vi "o3 49i Serial Data Recording & DECADEv3.1.vi"() -> ()   [LabVIEW 2014]
uses:
  <vilib>/Platform/TimedLoop/XDataNode/timing_clust.ctl
  <vilib>/Platform/TimedLoop/XDataNode/nitl_modes.ctl
  <vilib>/Platform/TimedLoop/XDataNode/wakeup.ctl
  C:/Program Files (x86)/National Instruments/LabVIEW 2014/examples/Data Communication/Network Streams/Simple Network Streams/support/Network Stream Command.ctl
  <vilib>/Utility/error.llb/whitespace.ctl
  <vilib>/Instr/_visa.llb/VISA Configure Serial Port (Instr).vi
  <vilib>/Utility/tcp.llb/UDP Multicast Write-Only Open.vi
  <vilib>/platform/TimedLoop/XDataNode/XDataNode.xnode
  <vilib>/Platform/TimedLoop/XDataNode/XDNodeRunTimeDep.lvlib
panel:
  out "Stop File Write":bool
  out "Default file name":string
  out "error out":errorcluster
  out "V6":bool
  in  "Clear Display\nErrors":bool
  out "Data Processing":bool
  out "Serial Visa Error":errorcluster
  out "SEPTIC TCP Error Out":errorcluster
  out "TCP packet\nSend to SEPTIC":bool
  out "UDP Time Stamp Offset":i32=1
  out "Data Array":string[](array[string])
  out "UDP packet \nstatus":bool
  out "UDP_Out_Error":errorcluster
  out "FISH TCP Error Out":errorcluster
  out "TCP packet\nSend to FISH":bool
  out "TCP Binary Packet":string
  out "Scan from String Error Counter\nfrom process loop":i32
  out "Read Error Counter\nfrom process loop":i32
  in  "milliseconds to wait":u32=330
  in  "ID":string="»"
  in  "VISA resource name":refnum<visa-resource-name>="ASRL6::INSTR"
  out "Data In Array":string[](array[string])
  out "UDP_ASCII_Out":string
  out "UDP_Pack_num":u32
  out "Flight Number":string
  in  "ue9LJ temp":u16
  out "Data String":string
  out "Internal packet":string[](array[string])
  out "RAW DATA":string
  in  "stop":bool
  out "Number of Send & Read Error\nfrom Acquire Loop":i32
  out "Command In":string
  # "o3_conc"
  # "Bench_temp"
  # "pressure"
  # "cell_a_nt"
  # "cell_b_int"
  # "flow_a"
  # "flow_b"
  # "lamp_temp"
  # "flags"
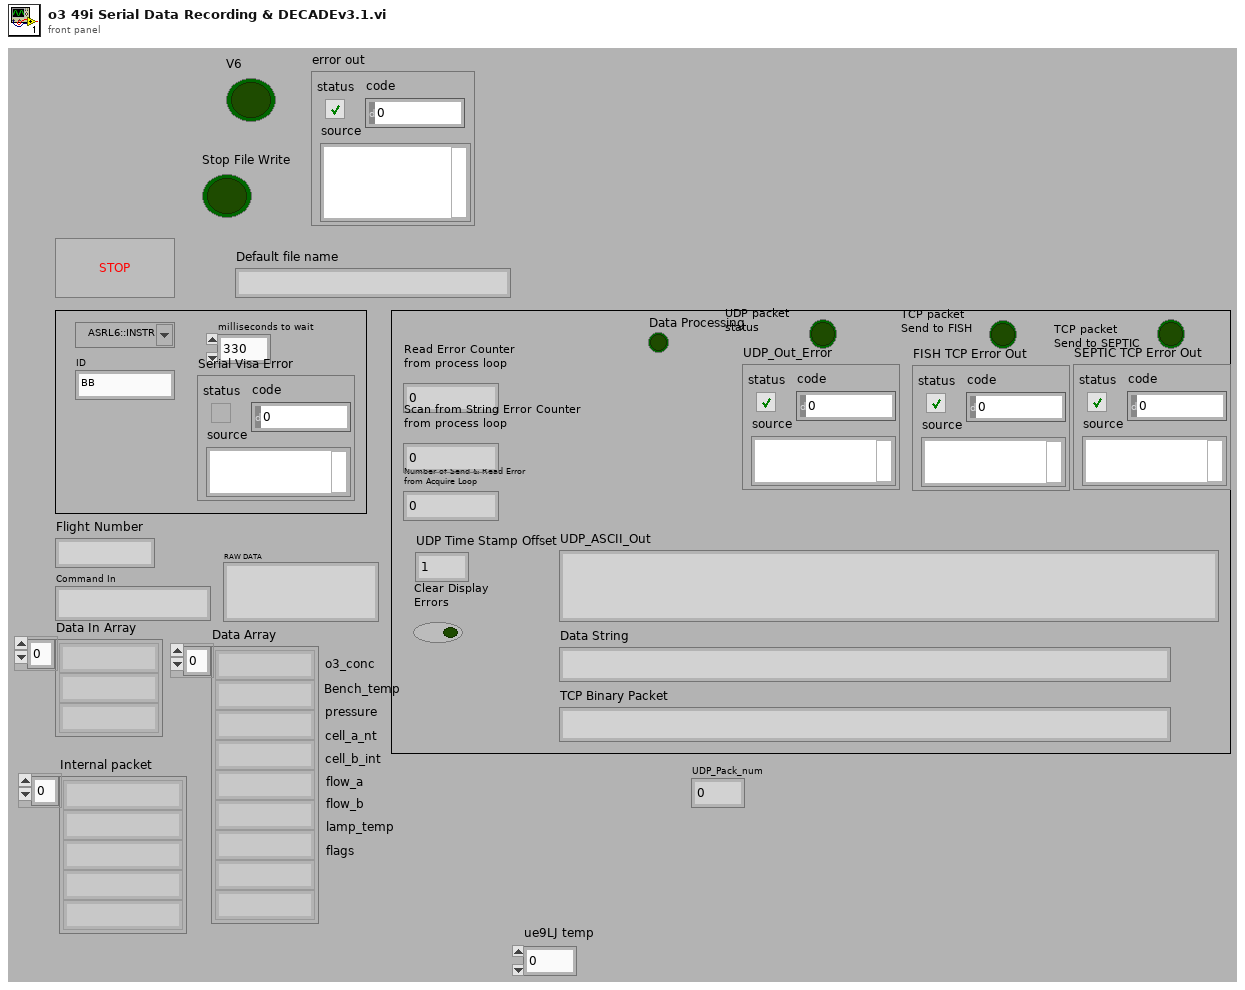
[diagram p1: front panel]
types:
  T1 = typedef "XDNodeRunTimeDep.lvlib/timing_clust.ctl" = cluster{"Expected End [f-1]":u64, "Actual End [f-1]":u64, "Finished Late? [f-1]":bool, "Expected End [i-1]":u64, "Actual End [i-1]":u64, "Finished Late? [i-1]":bool, "Expected Start [i]":u64, "Actual Start [i]":u64, "Expected Start [f]":u64, "Actual Start [f]":u64, "Source Name":string, "Structure Name":string, "Period":i64, "Deadline":i64, "Offset":i64, "Start":i64, "Priority":i32, "Timeout":i32, "Mode":T2, "Wakeup Reason":T3, "Error":errorcluster, "Source Type":string, "Secondary Source Type":string, "Global End Time":u64, "Global Start Time":u64, "Frame Duration":u64, "Iteration Duration":u64, "Assigned CPU":i32, "I/O Scan Engine Mode":u32}
  T2 = typedef "XDNodeRunTimeDep.lvlib/nitl_modes.ctl" = enum32{"No Change", "Process missed periods, maintain original phase", "Discard missed periods, maintain original phase", "Process missed periods, ignore original phase", "Discard missed periods, ignore original phase"}
  T3 = typedef "XDNodeRunTimeDep.lvlib/wakeup.ctl" = enum32{"Normal", "Aborted", "Asynchronous wakeup", "Timing source error", "Timed loop error", "Timeout"}
  T4 = typedef "Network Stream Command.ctl" = cluster{"Message":string, "Message Data":variant}
  T5 = enum16{"open", "replace", "create", "open or create", "replace or create", "replace or create with confirmation"}
  T6 = typedef "whitespace.ctl" = u16
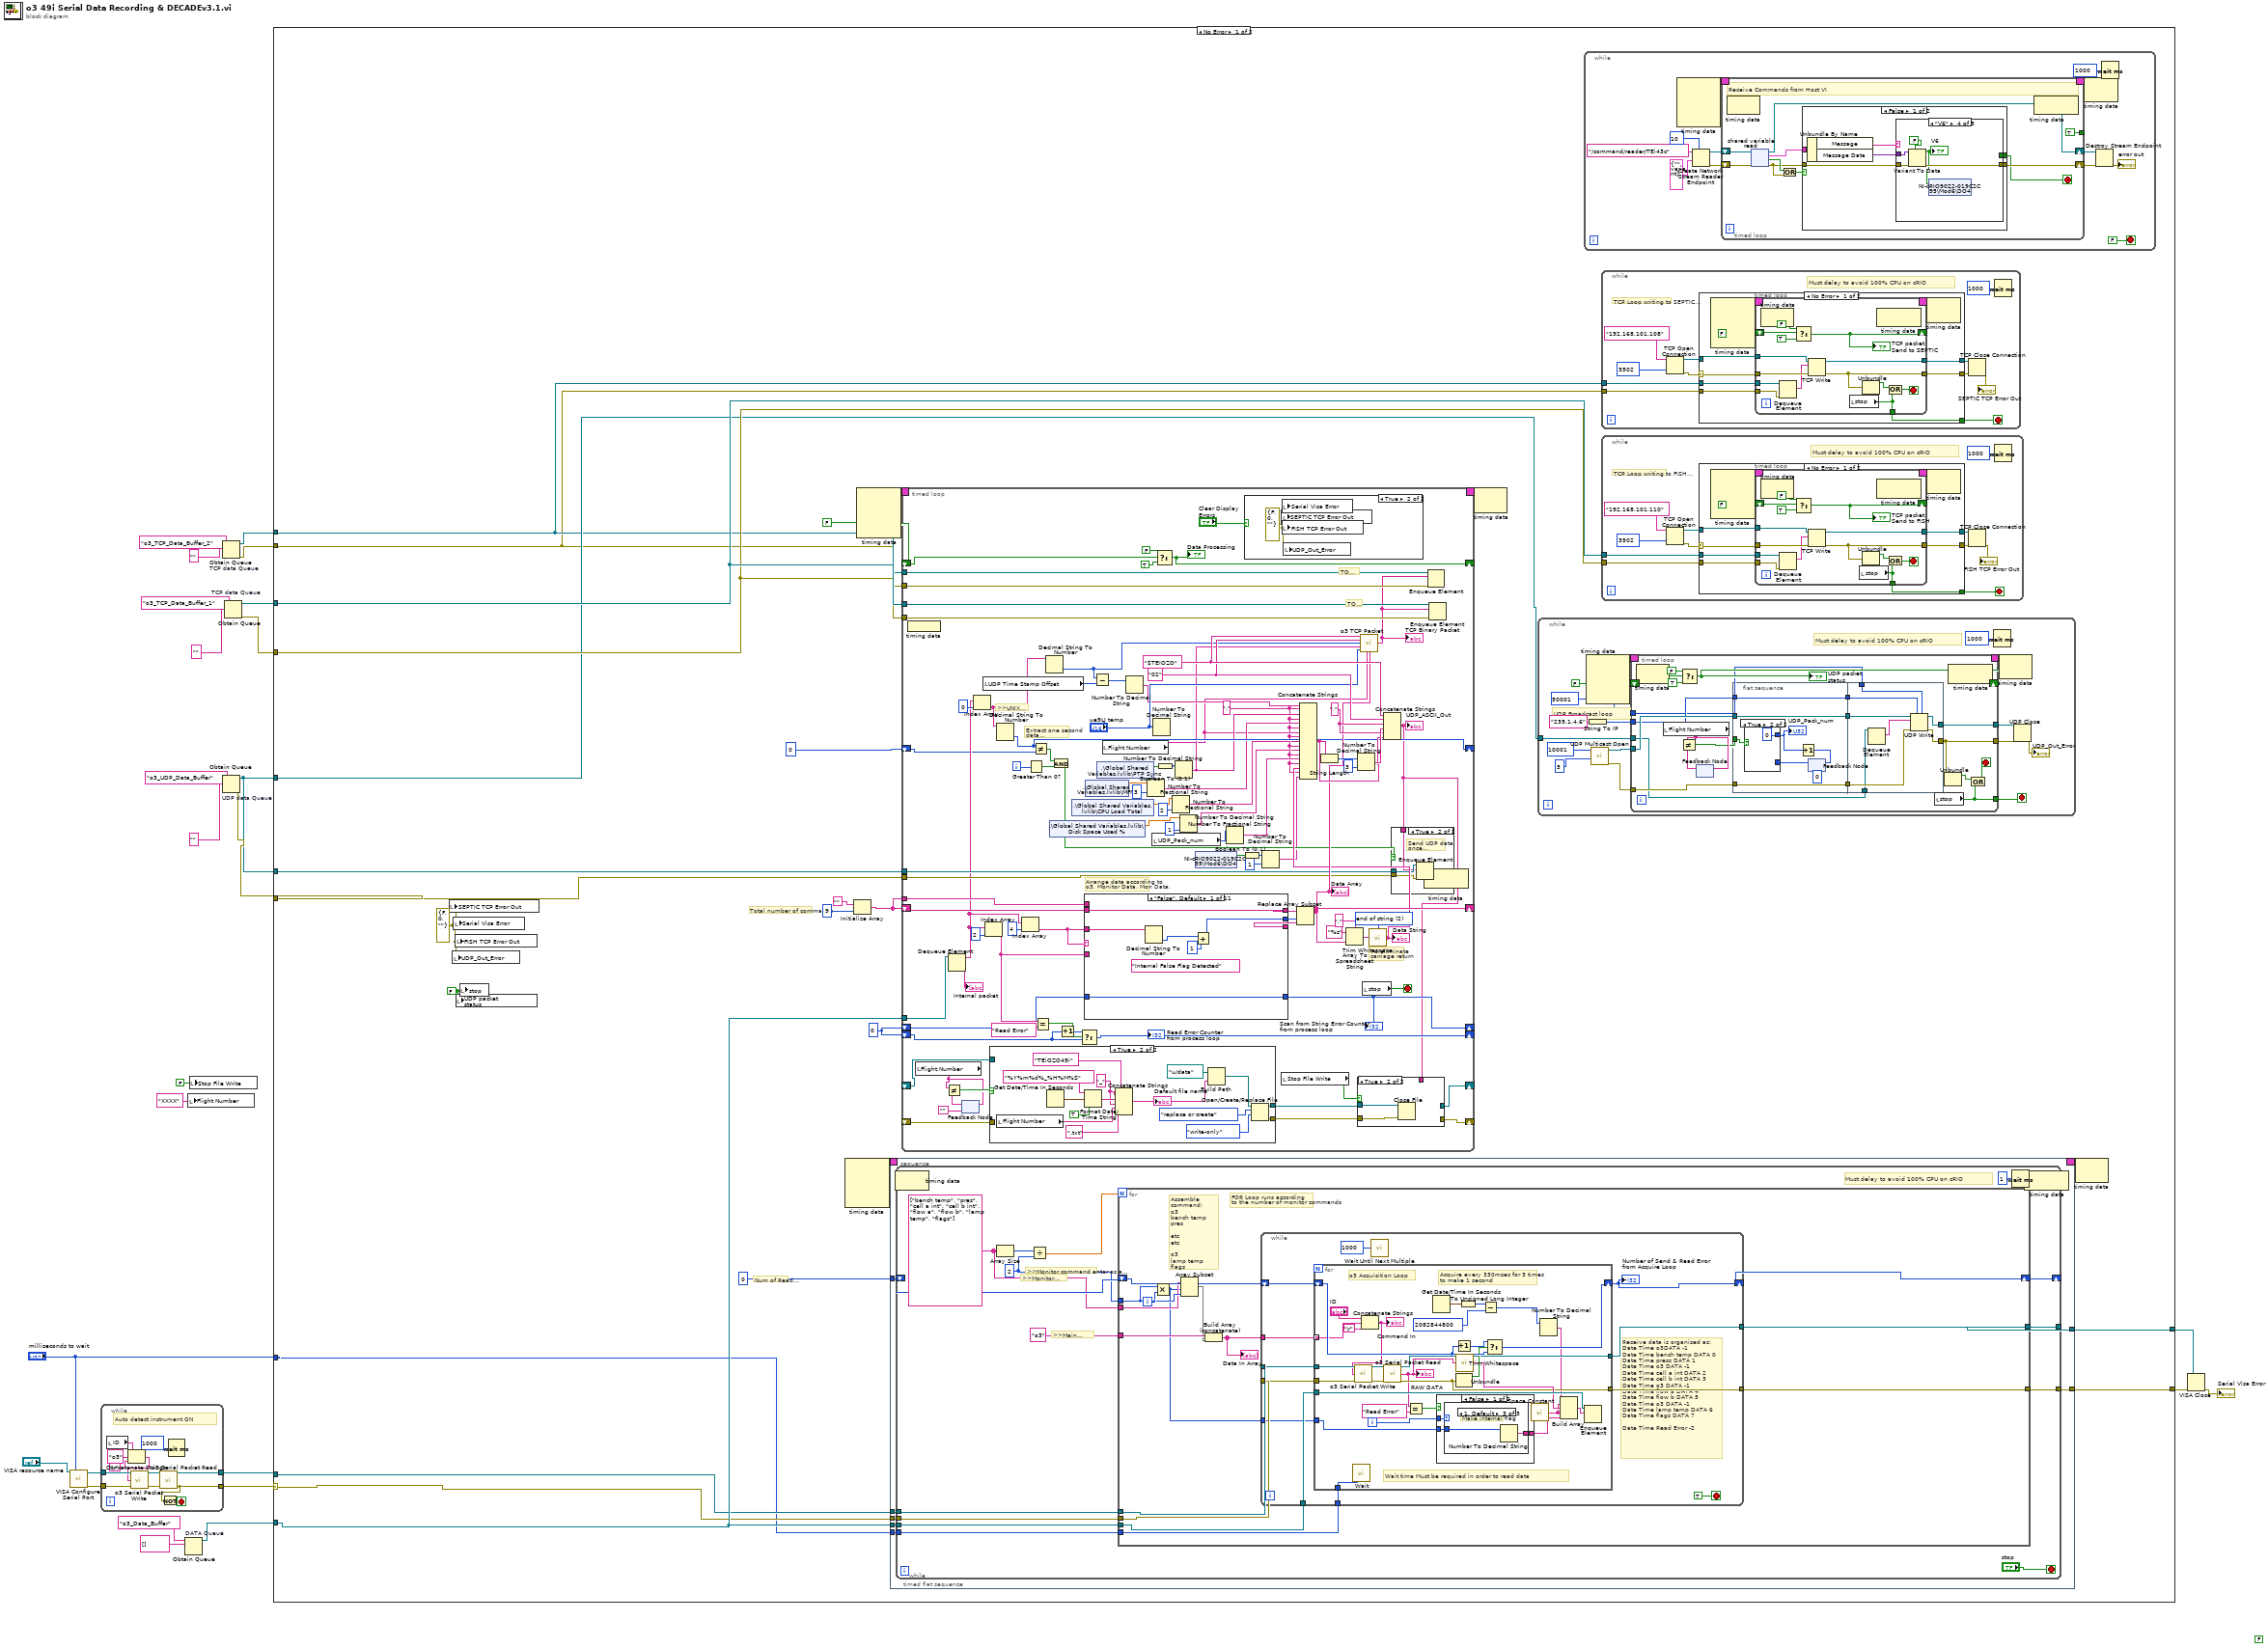
[diagram p0: block diagram]
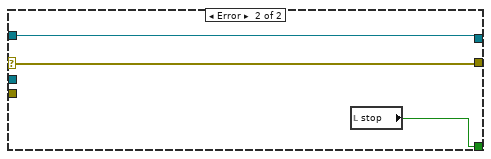
[diagram p2: hidden frame]
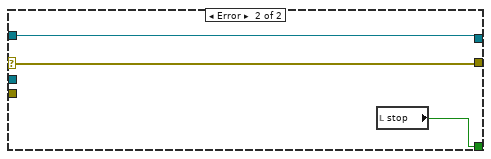
[diagram p3: hidden frame]
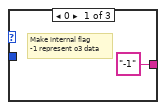
[diagram p4: hidden frame]
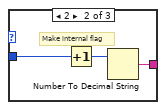
[diagram p5: hidden frame]
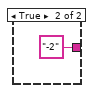
[diagram p6: hidden frame]
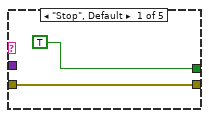
[diagram p7: hidden frame]
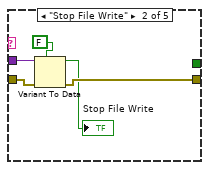
[diagram p8: hidden frame]
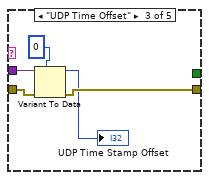
[diagram p9: hidden frame]
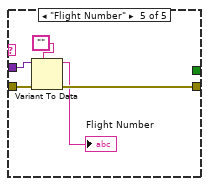
[diagram p10: hidden frame]
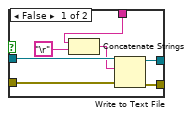
[diagram p14: hidden frame]
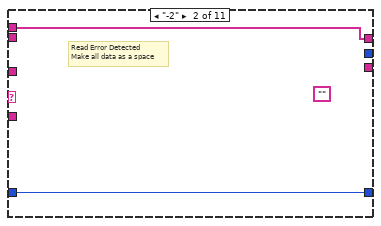
[diagram p17: hidden frame]
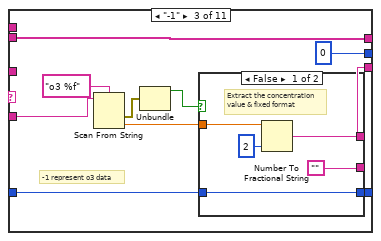
[diagram p18: hidden frame]
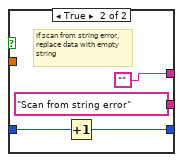
[diagram p19: hidden frame]
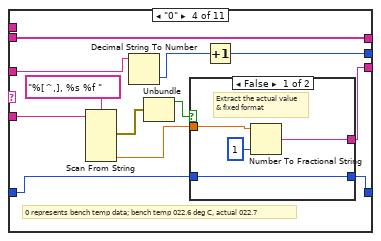
[diagram p20: hidden frame]
diagram:
  (unwired) FALSE
  n1 = call-poly "VISA Configure Serial Port"("VISA resource name"="VISA resource name", "timeout (10sec)"="milliseconds to wait") -> ("VISA resource name out"=w8:refnum<visa-resource-name>, "error out"=w7:errorcluster)  [unwired: 12 in]
  n2 = while {
    tunnel: [w36] -> w10
    tunnel: [w35] -> w9
    tunnel: w8 -> [w34]
    tunnel: w7 -> [w33]
    stop <- w37 stop-if-true
    # "Auto detect instrument ON"
    n3 = local read "ID"() -> (w31:string)
    n4 = Concatenate Strings(w31, "o3" ("string"), "\r") -> (w28:string)
    n5 = call "o3 Serial Packet Write.vi"("VISA resource name In"=w34, "Data in"=w28, "error in (no error)"=w33) -> ("VISA resource name Out"=w32:refnum<visa-resource-name>, "error out"=w38:errorcluster)  [unwired: 11 in]
    n6 = call "o3 Serial Packet Read.vi"("VISA resource In"=w32, "error in"=w38) -> ("VISA resource Out"=w35:refnum<visa-resource-name>, "error out"=w36:errorcluster)  [unwired: 11 in, 1 out]
    n7 = Not(x=w36) -> (.not. x?=w37:bool)
    n8 = Wait (ms)(milliseconds to wait=u32 1000) -> ()  [unwired: 1 out]
  }
  n9 = Obtain Queue "DATA Queue"(name (unnamed)="o3_Data_Buffer", element data type=string[] []) -> (queue out=w24:refnum<queue>)  [unwired: 3 in, 2 out]
  n10 = local write "Flight Number"("XXXX" ("Flight Number")) -> ()
  n11 = local write "Stop File Write"(FALSE ("Stop File Write")) -> ()
  n12 = Obtain Queue "TCP data Queue"(name (unnamed)="o3_TCP_Data_Buffer_2", element data type="") -> (queue out=w13:refnum<queue>, error out=w12:errorcluster)  [unwired: 3 in, 1 out]
  n13 = Obtain Queue "UDP data Queue"(name (unnamed)="o3_UDP_Data_Buffer", element data type="") -> (queue out=w14:refnum<queue>, error out=w15:errorcluster)  [unwired: 3 in, 1 out]
  n14 = Obtain Queue "TCP data Queue"(name (unnamed)="o3_TCP_Data_Buffer_1", element data type="") -> (queue out=w19:refnum<queue>, error out=w18:errorcluster)  [unwired: 3 in, 1 out]
  n15 = case shown="No Error" w10 {
    selector: w10 -> [w48 w678]
    tunnel: [w64 w678] -> w21
    tunnel: [w63 w677] -> w22
    tunnel: w24 -> [w60 _]
    tunnel: w9 -> [w47 w677]
    tunnel: w19 -> [w53 _]
    tunnel: w18 -> [w52 _]
    tunnel: w14 -> [w51 _]
    tunnel: w15 -> [w50 _]
    tunnel: w14 -> [w49 _]
    tunnel: w13 -> [w45 _]
    tunnel: w12 -> [w44 _]
    tunnel: "milliseconds to wait" -> [w43 _]
    frame No Error {
      w41 = errorcluster {"status"=FALSE, "code"=0, "source"=""} ("UDP Error Out")
      w55 = 0
      w54 = FALSE ("stop")
      # "Num of Read Error"
      # "Total number of commands"
      n16 = local write "SEPTIC TCP Error Out"(w41) -> ()
      n17 = local write "UDP_Out_Error"(w41) -> ()
      n18 = local write "Serial Visa Error"(w41) -> ()
      n19 = local write "FISH TCP Error Out"(w41) -> ()
      n20 = local write "UDP packet \nstatus"(w54) -> ()
      n21 = local write "stop"(w54) -> ()
      n22 = node-c288() -> (w40:T1)  [unwired: 4 in]
      n23 = Initialize Array("", 9) -> (w56:string[])
      n24 = node-c288() -> (w62:T1)  [unwired: 4 in]
      n25 = timed-sequence {
        timing: w40 -> [_]
        timing-out: [_] -> w39
        tunnel: [w155] -> w64
        tunnel: [w154] -> w63
        tunnel: w60 -> [w153]
        tunnel: 0 -> [w152]
        tunnel: w48 -> [w151]
        tunnel: w47 -> [w150]
        tunnel: w43 -> [w149]
        n26 = timed-flat-sequence {
          tunnel: [w162] -> w155
          tunnel: [w161] -> w154
          tunnel: w153 -> [w160]
          tunnel: w152 -> [w159]
          tunnel: w151 -> [w158]
          tunnel: w150 -> [w157]
          tunnel: w149 -> [w156]
          n27 = node-c288() -> ()  [unwired: 1 in, 1 out]
          n28 = while {
            tunnel: [w166] -> w162
            tunnel: w157 -> [w177]
            tunnel: w158 -> [w176]
            tunnel: [w175] -> w161
            tunnel: w160 -> [w174]
            shift-right: [w172] -> _
            shift-left: w159 -> [w173]
            tunnel: w156 -> [w164]
            stop <- "stop" stop-if-true
            w167 = 2
            w169 = string[] ["bench temp", "pres", "cell a int", "cell b int", "flow a", "flow b", "lamp temp", "flags"]
            # "Must delay to avoid 100% CPU on cRIO"
            # ">>Monitor command enter as a pair>>"
            # ">>Main commands>>"
            # ">>Monitor Command>>"
            n29 = Array Size(array=w169) -> (size(s)=w170:i32)
            n30 = Divide(x=w170, y=w167) -> (x/y=w168:dbl)
            n31 = for {
              N: w168 -> [_]
              tunnel: w177 -> [w185]
              tunnel: w176 -> [w184]
              tunnel: [w192] -> w166
              shift-right: [w190] -> w172
              shift-left: w173 -> [w191]
              tunnel: [w189] -> w175
              tunnel: w174 -> [w188]
              tunnel: w169 -> [w181]
              tunnel: "o3" -> [w186]
              tunnel: w167 -> [w182]
              tunnel: w164 -> [w178]
              i -> [w183]
              # "FOR Loop runs according\nto the number of monitor commands"
              # "Assemble command:\no3\nbench temp\npres\n\netc\netc\n\no3\nlamp temp\nflags"
              n32 = Multiply(x=w182, y=w183) -> (x*y=w179:i32)
              n33 = Array Subset(array=w181, index=w179, length=w182) -> (w180:string[])
              n34 = Build Array (concatenate)(w186, w180) -> (w187:string[])
              "Data In Array" <- w187
              n35 = while {
                tunnel: [w204] -> w192
                tunnel: w187 -> [w202]
                tunnel: [w200] -> w189
                tunnel: w188 -> [w199]
                tunnel: w184 -> [w198]
                tunnel: w185 -> [w197]
                tunnel: w179 -> [w196]
                shift-right: [w201] -> w190
                shift-left: w191 -> [w203]
                tunnel: w178 -> [w193]
                stop <- TRUE stop-if-true
                # "Receive data is organised as:\nDate Time o3DATA -1\nDate Time bench temp DATA 0\nDate Time press DATA 1\nDate Time o3 DATA -1\nDate Time cell a int DATA 2\nDate Time cell b int DATA 3\nDate Time o3 DATA -1\nDate Time flow a DATA 4\nDate Time flow b DATA 5\nDate Time o3 DATA -1\nDate Time lamp temp DATA 6\nDate Time flags DATA 7\n\nDate Time Read Error -2"
                n36 = for {
                  tunnel: w198 -> [w221]
                  tunnel: [w222] -> w204
                  tunnel: w202 -> [w219] mode=indexing
                  tunnel: [w223] -> w200
                  tunnel: w199 -> [w229]
                  tunnel: w197 -> [w224]
                  tunnel: w196 -> [w218]
                  shift-right: [w233] -> w201
                  shift-left: w203 -> [w234]
                  tunnel: w193 -> [w207]
                  i -> [w211]
                  # "Wait time Must be required in order to read data"
                  # "Acquire every 330msec for 3 times\nto make 1 second"
                  # "o3 Acquisition Loop"
                  n37 = call "Wait"("Count(mSec)"=w207) -> ()  [unwired: 1 out]
                  n38 = Concatenate Strings("ID", w219, "\r") -> (w217:string)
                  "Command In" <- w217
                  n39 = call "o3 Serial Packet Write.vi"("VISA resource name In"=w224, "Data in"=w217, "error in (no error)"=w221) -> ("VISA resource name Out"=w226:refnum<visa-resource-name>, "error out"=w225:errorcluster)  [unwired: 11 in]
                  n40 = call "o3 Serial Packet Read.vi"("VISA resource In"=w226, "error in"=w225) -> ("VISA resource Out"=w223:refnum<visa-resource-name>, "Data Out"=w214:string, "error out"=w222:errorcluster)  [unwired: 11 in]
                  "RAW DATA" <- w214
                  n41 = Equal?(x=w214, y="Read Error") -> (x = y?=w212:bool)
                  n42 = Get Date/Time In Seconds() -> (seconds since 1Jan1904=w206:timestamp)
                  n43 = case shown="False" w212 {
                    tunnel: [w237 "-2"] -> w227
                    tunnel: w211 -> [w236 _]
                    tunnel: w218 -> [w235 _]
                    frame False {
                      n44 = case shown="1, Default" w236 {
                        tunnel: ["-1" w241 w243] -> w237
                        tunnel: w235 -> [_ w239 w242]
                        frame 0 {
                          # "Make internal flag\n-1 represent o3 data"
                        }
                        frame 2 {
                          # "Make internal flag"
                          n45 = Increment(x=w239) -> (x+1=w240:i32)
                          n46 = Number To Decimal String(number=w240) -> (decimal integer string=w241:string)  [unwired: 1 in]
                        }
                        frame 1, Default {
                          # "Make internal flag"
                          n47 = Number To Decimal String(number=w242) -> (decimal integer string=w243:string)  [unwired: 1 in]
                        }
                      }
                    }
                    frame True {
                    }
                  }
                  n48 = Increment(x=w234) -> (x+1=w230:i32)
                  n49 = Unbundle(w222) -> ("status"=w231:bool)  [unwired: 2 out]
                  n50 = call <vilib>:"Trim Whitespace.vi"("string"=w214) -> ("trimmed string"=w228:string)  [unwired: 1 in]
                  n51 = To Unsigned Long Integer(number=w206) -> (unsigned 32bit integer=w210:u32)
                  n52 = Subtract(x=w210, y=u32 2082844800) -> (x-y=w205:u32)
                  n53 = Select(t=w230, s=w231, f=w234) -> (s? t:f=w233:i32)
                  n54 = call <vilib>:"Space Constant.vi"() -> ("String"=w215:string)
                  n55 = Number To Decimal String(number=w205) -> (decimal integer string=w208:string)  [unwired: 1 in]
                  n56 = Build Array(w208, w215, w228, w215, w227) -> (w216:string[])
                  n57 = Enqueue Element(queue=w229, element=w216) -> ()  [unwired: 2 in, 3 out]
                }
                "Number of Send & Read Error\nfrom Acquire Loop" <- w201
                n58 = call "Wait Until Next Multiple"("Count(mSec)"=u32 1000) -> ()  [unwired: 1 out]
              }
            }
            n59 = Wait (ms)(milliseconds to wait=u32 1) -> ()  [unwired: 1 out]
          }
          n60 = node-c288() -> ()  [unwired: 1 in, 1 out]
        }
      }
      n61 = timed-loop {
        timing: w62 -> [_]
        timing-out: [_] -> w61
        tunnel: w60 -> [w451]
        shift-right: [w419] -> _
        shift-left: w56 -> [w440]
        shift-right: [w428] -> _
        shift-left: w55 -> [w425]
        tunnel: w56 -> [w427]
        shift-right: [w423] -> _
        shift-left: w55 -> [w424]
        tunnel: w53 -> [w418]
        tunnel: w52 -> [w417]
        tunnel: w51 -> [w415]
        tunnel: w50 -> [w414]
        shift-right: [w406] -> _
        shift-left: 0 -> [w409]
        tunnel: w45 -> [w404]
        tunnel: w44 -> [w403]
        shift-right: [w395] -> _
        shift-left: FALSE -> [w398]
        shift-right: [w392] -> _
        shift-left: _ -> [w384]
        shift-right: [w382] -> _
        shift-left: _ -> [w383]
        i -> [w407]
        stop <- w449 stop-if-true
        w433 = T6 2 items=["both", "start of string", "end of string"] ("location (both)")
        w369 = ","
        w421 = "02"
        w442 = ","
        w422 = "$TEIOZO"
        # "TO SEPTIC"
        # "TO FISH"
        # "Extract one second data\nfor UDP sending"
        # "Arrange data according to\no3, Monitor Data, Mon Data,"
        # "To eliminate\ncarriage return"
        # ">>UNIX TIME>>"
        n62 = node-c288() -> ()  [unwired: 1 in]
        n63 = local read "Flight Number"() -> (w387:string)
        n64 = Dequeue Element(queue=w451) -> (element=w412:string[])  [unwired: 2 in, 3 out]
        "Internal packet" <- w412
        n65 = feedback #1("" ("Flight Number")) -> (w389:string)
        n66 = Not Equal?(x=w387, y=w389) -> (x != y?=w388:bool)
        n67 = feedback-in #1(w387) -> ()
        n68 = Index Array(array=w412, index=0) -> (element=w411:string)
        n69 = local read "UDP Time Stamp Offset"() -> (w364:i32)
        n70 = Index Array(array=w412, index=2) -> (element=w431:string)
        n71 = case shown="True" w388 {
          tunnel: [w453 w455] -> w386
          tunnel: [w452 w454] -> w385
          tunnel: w384 -> [w453 _]
          tunnel: w383 -> [w452 _]
          frame False {
          }
          frame True {
            w462 = "_" ("string")
            n72 = local read "Flight Number"() -> (w468:string)
            n73 = Get Date/Time In Seconds() -> (seconds since 1Jan1904=w463:timestamp)
            n74 = Format Date/Time String(time format string (%c)="%Y%m%d%_%H%M%S", seconds (now)=w463, UTC format=TRUE) -> (date/time string=w466:string)
            n75 = Concatenate Strings("TEiOZO49i" ("string"), w462, w466, w462, w468, ".txt" ("string")) -> (w460:string)
            "Default file name" <- w460
            n76 = Build Path(base path=path "u:/data", name or relative path=w460) -> (appended path=w456:path)
            n77 = Open/Create/Replace File(file path (use dialog)=w456, operation (0:open)=T5."replace or create", access (0:read/write)=enum16{"read/write", "read-only", "write-only"}."write-only") -> (refnum out=w455:refnum<file>, error out=w454:errorcluster)  [unwired: 3 in, 1 out]
          }
        }
        n78 = Decimal String To Number(string=w411) -> (number=w406:i32)  [unwired: 2 in, 1 out]
        n79 = Index Array(array=w412, index=4) -> (element=w439:string)
        n80 = Greater Than 0?(x=w407) -> (x > 0?=w410:bool)
        n81 = Not Equal?(x=w406, y=w409) -> (x != y?=w408:bool)
        n82 = Equal?(x=w431, y="Read Error") -> (x = y?=w429:bool)
        n83 = Decimal String To Number(string=w411) -> (number=w400:i32)  [unwired: 2 in, 1 out]
        n84 = shared-variable ".\\Global Shared Variables.lvlib\\Disk Space Used %"() -> (w366:dbl)  [unwired: 1 in, 1 out]
        n85 = Compound Arithmetic op=AND(w408, w410) -> (w405:bool)
        n86 = Increment(x=w425) -> (x+1=w426:i32)
        n87 = shared-variable ".\\Global Shared Variables.lvlib\\CPU Load Total"() -> (w381:dbl)  [unwired: 1 in, 1 out]
        n88 = Select(t=w426, s=w429, f=w425) -> (s? t:f=w428:i32)
        "Read Error Counter\nfrom process loop" <- w428
        n89 = case shown="\"False\", Default" w439 {
          tunnel: w439 -> [w486 _ _ w519 w538 w559 w580 w601 w622 w643 w664]
          tunnel: w440 -> [w487 _ w499 w520 w539 w560 w581 w602 w623 w644 w665]
          tunnel: w431 -> [_ _ w496 w515 w534 w556 w577 w598 w619 w640 w661]
          tunnel: [w487 w489 w499 w520 w539 w560 w581 w602 w623 w644 w665] -> w438
          tunnel: [w484 _ 0 ("index") w517 w536 w557 w578 w599 w620 w641 w662] -> w437
          tunnel: [_ _ w494 w513 w532 w555 w576 w597 w618 w639 w656] -> w436
          tunnel: w427 -> [_ w489 _ _ _ _ _ _ _ _ _]
          tunnel: w424 -> [w482 w488 w491 w510 w529 w550 w571 w592 w613 w634 w655]
          tunnel: [w482 w488 w490 w509 w528 w549 w570 w591 w612 w633 w654] -> w423
          frame "False", Default {
            (unwired) "Internal False Flag Detected"
            n90 = Decimal String To Number(string=w486) -> (number=w483:i32)  [unwired: 2 in, 1 out]
            n91 = Add(x=w483, y=1) -> (x+y=w484:i32)
          }
          frame "-2" {
            (unwired) ""
            # "Read Error Detected\nMake all data as a space"
          }
          frame "-1" {
            # "-1 represent o3 data"
            n92 = Scan From String(format string="o3 %f", input string=w496) -> (error out=w493:errorcluster, output 1=w495:dbl)  [unwired: 3 in, 2 out]
            n93 = Unbundle(w493) -> ("status"=w492:bool)  [unwired: 2 out]
            n94 = case shown="False" w492 {
              tunnel: w495 -> [w504 _]
              tunnel: [w503 ""] -> w494
              tunnel: w491 -> [w502 w507]
              tunnel: [w502 w506] -> w490
              tunnel: ["" "Scan from string error"] -> _
              frame False {
                # "Extract the concentration\nvalue & fixed format"
                n95 = Number To Fractional String(number=w504, precision (6)=i16 2) -> (F-format string=w503:string)  [unwired: 2 in]
              }
              frame True {
                # "If scan from string error,\nreplace data with empty\nstring"
                n96 = Increment(x=w507) -> (x+1=w506:i32)
              }
            }
          }
          frame "0" {
            # "0 represents bench temp data; bench temp 022.6 deg C, actual 022.7"
            n97 = Scan From String(format string="%[^,], %s %f ", input string=w515) -> (error out=w512:errorcluster, output 3=w514:dbl)  [unwired: 7 in, 2 out]
            n98 = Decimal String To Number(string=w519) -> (number=w518:i32)  [unwired: 2 in, 1 out]
            n99 = Unbundle(w512) -> ("status"=w511:bool)  [unwired: 2 out]
            n100 = case shown="False" w511 {
              tunnel: w514 -> [w524 _]
              tunnel: [w523 ""] -> w513
              tunnel: w510 -> [w522 w526]
              tunnel: [w522 w525] -> w509
              frame False {
                # "Extract the actual value\n& fixed format"
                n101 = Number To Fractional String(number=w524, precision (6)=i16 1) -> (F-format string=w523:string)  [unwired: 2 in]
              }
              frame True {
                (unwired) "Scan from string error"
                # "If scan from string error,\nreplace data with empty\nstring"
                n102 = Increment(x=w526) -> (x+1=w525:i32)
              }
            }
            n103 = Increment(x=w518) -> (x+1=w517:i32)
          }
          frame "1" {
            # "1 represents pres data; pres 725.3 mmHg, actual 725.4"
            n104 = Scan From String(format string="%[^,], %s %f ", input string=w534) -> (error out=w531:errorcluster, output 3=w533:dbl)  [unwired: 7 in, 2 out]
            n105 = Decimal String To Number(string=w538) -> (number=w537:i32)  [unwired: 2 in, 1 out]
            n106 = Unbundle(w531) -> ("status"=w530:bool)  [unwired: 2 out]
            n107 = case shown="False" w530 {
              tunnel: w533 -> [w544 _]
              tunnel: [w543 ""] -> w532
              tunnel: w529 -> [w542 w547]
              tunnel: [w542 w546] -> w528
              tunnel: ["" "Scan from string error"] -> _
              frame False {
                # "Extract the actual value\n& fixed format"
                n108 = Number To Fractional String(number=w544, precision (6)=i16 1) -> (F-format string=w543:string)  [unwired: 2 in]
              }
              frame True {
                # "If scan from string error,\nreplace data with empty\nstring"
                n109 = Increment(x=w547) -> (x+1=w546:i32)
              }
            }
            n110 = Increment(x=w537) -> (x+1=w536:i32)
          }
          frame "2" {
            # "2 represents cell a int data; cell a int 63246 Hz"
            n111 = Scan From String(format string="cell a int %d", input string=w556) -> (error out=w552:errorcluster, output 1=w553:i32)  [unwired: 3 in, 2 out]
            n112 = Decimal String To Number(string=w559) -> (number=w558:i32)  [unwired: 2 in, 1 out]
            n113 = Unbundle(w552) -> ("status"=w551:bool)  [unwired: 2 out]
            n114 = case shown="False" w551 {
              tunnel: [w565 ""] -> w555
              tunnel: w553 -> [w564 _]
              tunnel: w550 -> [w563 w568]
              tunnel: [w563 w567] -> w549
              tunnel: ["" "Scan from string error"] -> _
              frame False {
                # "Extract the actual value\n& fixed format"
                n115 = Number To Fractional String(number=w564, precision (6)=i16 0) -> (F-format string=w565:string)  [unwired: 2 in]
              }
              frame True {
                # "If scan from string error,\nreplace data with empty\nstring"
                n116 = Increment(x=w568) -> (x+1=w567:i32)
              }
            }
            n117 = Increment(x=w558) -> (x+1=w557:i32)
          }
          frame "3" {
            # "3 represents cell b int data; cell b int 63246 Hz"
            n118 = Scan From String(format string="cell b int %d", input string=w577) -> (error out=w573:errorcluster, output 1=w574:i32)  [unwired: 3 in, 2 out]
            n119 = Decimal String To Number(string=w580) -> (number=w579:i32)  [unwired: 2 in, 1 out]
            n120 = Unbundle(w573) -> ("status"=w572:bool)  [unwired: 2 out]
            n121 = case shown="False" w572 {
              tunnel: [w586 ""] -> w576
              tunnel: w574 -> [w585 _]
              tunnel: w571 -> [w584 w589]
              tunnel: [w584 w588] -> w570
              tunnel: ["" "Scan from string error"] -> _
              frame False {
                # "Extract the actual value\n& fixed format"
                n122 = Number To Fractional String(number=w585, precision (6)=i16 0) -> (F-format string=w586:string)  [unwired: 2 in]
              }
              frame True {
                # "If scan from string error,\nreplace data with empty\nstring"
                n123 = Increment(x=w589) -> (x+1=w588:i32)
              }
            }
            n124 = Increment(x=w579) -> (x+1=w578:i32)
          }
          frame "4" {
            # "4 represents flow a data; flow a 0.696 l/m"
            n125 = Scan From String(format string="flow a %f", input string=w598) -> (error out=w594:errorcluster, output 1=w595:dbl)  [unwired: 3 in, 2 out]
            n126 = Decimal String To Number(string=w601) -> (number=w600:i32)  [unwired: 2 in, 1 out]
            n127 = Unbundle(w594) -> ("status"=w593:bool)  [unwired: 2 out]
            n128 = case shown="False" w593 {
              tunnel: [w607 ""] -> w597
              tunnel: w595 -> [w606 _]
              tunnel: w592 -> [w605 w610]
              tunnel: [w605 w609] -> w591
              tunnel: ["" "Scan from string error"] -> _
              frame False {
                # "Extract the actual value\n& fixed format"
                n129 = Number To Fractional String(number=w606, precision (6)=i16 3) -> (F-format string=w607:string)  [unwired: 2 in]
              }
              frame True {
                # "If scan from string error,\nreplace data with empty\nstring"
                n130 = Increment(x=w610) -> (x+1=w609:i32)
              }
            }
            n131 = Increment(x=w600) -> (x+1=w599:i32)
          }
          frame "5" {
            # "5 represents flow b data; flow b 0.696 l/m"
            n132 = Scan From String(format string="flow b %f", input string=w619) -> (error out=w615:errorcluster, output 1=w616:dbl)  [unwired: 3 in, 2 out]
            n133 = Decimal String To Number(string=w622) -> (number=w621:i32)  [unwired: 2 in, 1 out]
            n134 = Unbundle(w615) -> ("status"=w614:bool)  [unwired: 2 out]
            n135 = case shown="False" w614 {
              tunnel: [w628 ""] -> w618
              tunnel: w616 -> [w627 _]
              tunnel: w613 -> [w626 w631]
              tunnel: [w626 w630] -> w612
              tunnel: ["" "Scan from string error"] -> _
              frame False {
                # "Extract the actual value\n& fixed format"
                n136 = Number To Fractional String(number=w627, precision (6)=i16 3) -> (F-format string=w628:string)  [unwired: 2 in]
              }
              frame True {
                # "If scan from string error,\nreplace data with empty\nstring"
                n137 = Increment(x=w631) -> (x+1=w630:i32)
              }
            }
            n138 = Increment(x=w621) -> (x+1=w620:i32)
          }
          frame "6" {
            # "6 represents lamp temp data; lamp temp 056.1 deg C"
            n139 = Scan From String(format string="lamp temp %f", input string=w640) -> (error out=w636:errorcluster, output 1=w637:dbl)  [unwired: 3 in, 2 out]
            n140 = Decimal String To Number(string=w643) -> (number=w642:i32)  [unwired: 2 in, 1 out]
            n141 = Unbundle(w636) -> ("status"=w635:bool)  [unwired: 2 out]
            n142 = case shown="False" w635 {
              tunnel: [w649 ""] -> w639
              tunnel: w637 -> [w648 _]
              tunnel: w634 -> [w647 w652]
              tunnel: [w647 w651] -> w633
              tunnel: ["" "Scan from string error"] -> _
              frame False {
                # "Extract the actual value\n& fixed format"
                n143 = Number To Fractional String(number=w648, precision (6)=i16 1) -> (F-format string=w649:string)  [unwired: 2 in]
              }
              frame True {
                # "If scan from string error,\nreplace data with empty\nstring"
                n144 = Increment(x=w652) -> (x+1=w651:i32)
              }
            }
            n145 = Increment(x=w642) -> (x+1=w641:i32)
          }
          frame "7" {
            # "7 represents flags data; flags 1c100000"
            n146 = Scan From String(format string="flags %s", input string=w661) -> (error out=w659:errorcluster, output 1=w657:string)  [unwired: 3 in, 2 out]
            n147 = Decimal String To Number(string=w664) -> (number=w663:i32)  [unwired: 2 in, 1 out]
            n148 = Unbundle(w659) -> ("status"=w658:bool)  [unwired: 2 out]
            n149 = case shown="False" w658 {
              tunnel: w657 -> [w668 _]
              tunnel: [w668 ""] -> w656
              tunnel: w655 -> [w667 w671]
              tunnel: [w667 w670] -> w654
              tunnel: ["" "Scan from string error"] -> _
              frame False {
                # "Extract the actual value\n& fixed format"
              }
              frame True {
                # "If scan from string error,\nreplace data with empty\nstring"
                n150 = Increment(x=w671) -> (x+1=w670:i32)
              }
            }
            n151 = Increment(x=w663) -> (x+1=w662:i32)
          }
        }
        "Scan from String Error Counter\nfrom process loop" <- w423
        n152 = shared-variable ".\\Global Shared Variables.lvlib\\MFM"() -> (w380:dbl)  [unwired: 1 in, 1 out]
        n153 = Subtract(x=w400, y=w364) -> (x-y=w401:i32)
        n154 = shared-variable ".\\Global Shared Variables.lvlib\\PTP Sync"() -> (w376:bool)  [unwired: 1 in, 1 out]
        n155 = local read "Flight Number"() -> (w370:string)
        n156 = Number To Decimal String(number=w401) -> (decimal integer string=w399:string)  [unwired: 1 in]
        n157 = Number To Fractional String(number=w380, precision (6)=i16 3) -> (F-format string=w375:string)  [unwired: 2 in]
        n158 = local read "UDP_Pack_num"() -> (w447:u32)
        n159 = Number To Decimal String(number="ue9LJ temp") -> ()  [unwired: 1 in, 1 out]
        n160 = Select(t=FALSE, s=w398, f=TRUE) -> (s? t:f=w395:bool)
        "Data Processing" <- w395
        n161 = Boolean To (0,1)(Boolean=w376) -> (0, 1=w377:i16)
        n162 = Number To Fractional String(number=w381, precision (6)=i16 2) -> (F-format string=w368:string)  [unwired: 2 in]
        n163 = Number To Decimal String(number=w377) -> (decimal integer string=w371:string)  [unwired: 1 in]
        n164 = Number To Fractional String(number=w366, precision (6)=i16 1) -> (F-format string=w365:string)  [unwired: 2 in]
        n165 = shared-variable "NI-cRIO9022-019C2C95\\Mod6\\DO4"() -> (w372:bool)  [unwired: 1 in, 1 out]
        n166 = Number To Decimal String(number=w447) -> (decimal integer string=w446:string)  [unwired: 1 in]
        n167 = Boolean To (0,1)(Boolean=w372) -> (0, 1=w374:i16)
        n168 = case shown="True" "Clear Display\nErrors" {
          frame False {
          }
          frame True {
            w478 = errorcluster {"status"=FALSE, "code"=0, "source"=""} ("UDP Error Out")
            n169 = local write "SEPTIC TCP Error Out"(w478) -> ()
            n170 = local write "Serial Visa Error"(w478) -> ()
            n171 = local write "FISH TCP Error Out"(w478) -> ()
            n172 = local write "UDP_Out_Error"(w478) -> ()
          }
        }
        n173 = Number To Decimal String(number=w374, width (-)=i16 1) -> (decimal integer string=w373:string)
        n174 = local read "Stop File Write"() -> (w391:bool)
        n175 = Replace Array Subset(array=w438, new element=w436, index=w437) -> (w419:string[])
        "Data Array" <- w419
        n176 = Array To Spreadsheet String(delimiter (Tab)=",", array=w419, 3:"%s" ("format string")) -> (spreadsheet string=w432:string)
        n177 = call "o3 TCP Packet.vi"("ID"=w422, "Version"=w421, "utc_time"=w400, "PTP Sync"=w371, "ue9LJ temp"="ue9LJ temp", "Flight Number"=w370, "Data Array"=w419) -> ("TCP Binary Packet"=w402:string)  [unwired: 8 in]
        "TCP Binary Packet" <- w402
        n178 = local read "stop"() -> (w449:bool)
        n179 = call <vilib>:"Trim Whitespace.vi"("string"=w432, "location (both)"=w433) -> ("trimmed string"=w416:string)
        "Data String" <- w416
        n180 = Concatenate Strings(w399, w369, w371, w369, w375, w369, w370, w369, w368, w369, w365, w369, w446, w369, w416, w369, w373) -> (w441:string)
        n181 = String Length(string=w441) -> (length=w445:i32)
        n182 = Number To Decimal String(number=w445, width (-)=i16 3) -> (decimal integer string=w443:string)
        n183 = Concatenate Strings(w422, w421, w442, w443, w442, w441) -> (w393:string)
        "UDP_ASCII_Out" <- w393
        n184 = case shown="True" w391 {
          tunnel: w386 -> [w475 w477]
          tunnel: w385 -> [w474 w476]
          tunnel: [w471 _] -> w392
          tunnel: w393 -> [w470 _]
          tunnel: [w469 _] -> w382
          frame False {
            n185 = Concatenate Strings(w470, "\r") -> (w472:string)
            n186 = Write to Text File(file (use dialog)=w475, text=w472, error in=w474) -> (refnum out=w471:refnum<file>, error out=w469:errorcluster)  [unwired: 2 out]
          }
          frame True {
            n187 = Close File(refnum=w477, error in=w476) -> ()  [unwired: 2 out]
          }
        }
        n188 = case shown="True" w405 {
          tunnel: w415 -> [_ w481]
          tunnel: w414 -> [_ w480]
          tunnel: w393 -> [_ w479]
          frame False {
          }
          frame True {
            # "Send UDP data once\na second"
            n189 = Enqueue Element(queue=w481, element=w479, error in (no error)=w480) -> ()  [unwired: 1 in, 3 out]
          }
        }
        n190 = node-c288() -> ()  [unwired: 1 in, 1 out]
        n191 = Enqueue Element(queue=w404, element=w402, error in (no error)=w403) -> ()  [unwired: 1 in, 3 out]
        n192 = Enqueue Element(queue=w418, element=w402, error in (no error)=w417) -> ()  [unwired: 1 in, 3 out]
      }
      n193 = node-c288(w61) -> ()  [unwired: 1 out]
      n194 = while {
        tunnel: w49 -> [w306]
        stop <- w307 stop-if-true
        # "Must delay to avoid 100% CPU on cRIO"
        # "UDP Broadcast loop"
        n195 = node-c288() -> (w309:T1)  [unwired: 4 in]
        n196 = String To IP(1:"239.1.4.6" ("name")) -> (0:w311:u32)
        n197 = call-poly <vilib>:"UDP Multicast Open.vi"("time-to-live (1)"=u16 5, "port"=u16 10001) -> ("error out"=w319:errorcluster, "connection ID"=w320:refnum<k16>)  [unwired: 8 in]
        n198 = timed-loop {
          tunnel: w320 -> [w340]
          tunnel: w319 -> [w339]
          tunnel: [w326] -> w315
          shift-right: [w329] -> _
          shift-left: FALSE -> [w332]
          tunnel: [w324] -> w313
          tunnel: w311 -> [w328]
          tunnel: u16 50001 ("port or service name") -> [w327]
          timing: w309 -> [_]
          timing-out: [_] -> w308
          tunnel: [w322] -> w307
          tunnel: w306 -> [w321]
          stop <- w323 stop-if-true
          n199 = node-c288() -> ()  [unwired: 1 in, 1 out]
          n200 = local read "Flight Number"() -> (w335:string)
          n201 = Select(t=FALSE, s=w332, f=TRUE) -> (s? t:f=w329:bool)
          "UDP packet \nstatus" <- w329
          n202 = feedback-in #2(w335) -> ()
          n203 = feedback #2() -> (w334:string)  [unwired: 1 in]
          n204 = Not Equal?(x=w335, y=w334) -> (x != y?=w333:bool)
          n205 = flat-sequence {
            tunnel: w328 -> [w348]
            tunnel: w339 -> [w349]
            tunnel: w340 -> [w350]
            tunnel: [w350] -> w338
            tunnel: [w349] -> w337
            tunnel: [w348] -> w336
            tunnel: w333 -> [w347]
            tunnel: w327 -> [w360]
            tunnel: w338 -> [w359]
            tunnel: w337 -> [w358]
            tunnel: w336 -> [w357]
            tunnel: [w356] -> w326
            tunnel: [w355] -> w324
            tunnel: w321 -> [w354]
            frame #0 {
              n206 = feedback #3(u32 0) -> (w344:u32)
              n207 = case shown="True" w347 {
                tunnel: w344 -> [w351 _]
                tunnel: [w351 u32 0] -> w343
                frame False {
                }
                frame True {
                }
              }
              "UDP_Pack_num" <- w343
              n208 = Increment(x=w343) -> (x+1=w345:u32)
              n209 = feedback-in #3(w345) -> ()
            }
            frame #1 {
              n210 = Dequeue Element(queue=w354) -> (element=w353:string)  [unwired: 2 in, 3 out]
              n211 = UDP Write(address=w357, port or service name=w360, connection ID=w359, data in=w353, 8:w358) -> (error out=w355:errorcluster, 3:w356:refnum<k16>)  [unwired: 1 in]
            }
          }
          n212 = local read "stop"() -> (w322:bool)
          n213 = Unbundle(w324) -> ("status"=w325:bool)  [unwired: 2 out]
          n214 = node-c288() -> ()  [unwired: 1 in, 1 out]
          n215 = Compound Arithmetic op=OR(w325, w322) -> (w323:bool)
        }
        n216 = Wait (ms)(milliseconds to wait=u32 1000) -> ()  [unwired: 1 out]
        n217 = node-c288(w308) -> ()  [unwired: 1 out]
        n218 = UDP Close(connection ID=w315, 8:w313) -> (error out=→"UDP_Out_Error":errorcluster)  [unwired: 1 out]
      }
      n219 = while {
        stop <- FALSE stop-if-true
        n220 = node-c288() -> (w250:T1)  [unwired: 4 in]
        n221 = Create Network Stream Reader Endpoint(7:10 ("reader buffer size"), 9:T4 {"Message"="", "Message Data"=variant} ("Message Cluster"), 11:"/command/reader/TEi43c" ("reader url")) -> (0:w256:errorcluster, 3:w257:refnum<k21>)  [unwired: 4 in]
        n222 = timed-loop "Host->Target Command Reader" {
          shift-right: [w267] -> w254
          shift-left: w256 -> [w270]
          shift-right: [w268] -> w253
          shift-left: w257 -> [w269]
          tunnel: [TRUE] -> _
          timing: w250 -> [_]
          timing-out: [_] -> w249
          stop <- w261 stop-if-true
          # "Receive Commands from Host VI"
          n223 = node-c288() -> ()  [unwired: 1 in, 1 out]
          n224 = shared-variable-read(w269, w270) -> (w268:refnum<k21>, w263:errorcluster, w265:bool, w266:T4)  [unwired: 1 in]
          n225 = Or(x=w265, y=w263) -> (x .or. y?=w264:bool)
          n226 = case shown="False" w264 {
            selector: w264 -> [_ w301]
            tunnel: w263 -> [w278 w302]
            tunnel: [w277 w302] -> w267
            tunnel: w266 -> [w275 _]
            tunnel: [w276 w301] -> w261
            frame False {
              n227 = Unbundle By Name(w275) -> ("Message"=w274:string, "Message Data"=w273:variant)
              n228 = case shown="\"V6\"" w274 {
                tunnel: w278 -> [w280 w284 w289 w295 w300]
                tunnel: [w280 w282 w288 w294 w299] -> w277
                tunnel: w273 -> [_ w285 w290 w293 w298]
                tunnel: [TRUE _ _ _ _] -> w276
                frame "Stop", Default {
                }
                frame "Stop File Write" {
                  n229 = Variant To Data(error in=w284, type=FALSE, Variant=w285) -> (data=→"Stop File Write":bool, error out=w282:errorcluster)
                }
                frame "UDP Time Offset" {
                  n230 = Variant To Data(error in=w289, type=0, Variant=w290) -> (data=→"UDP Time Stamp Offset":i32, error out=w288:errorcluster)
                }
                frame "V6" {
                  n231 = Variant To Data(error in=w295, type=FALSE, Variant=w293) -> (data=w291:bool, error out=w294:errorcluster)
                  "V6" <- w291
                  n232 = shared-variable "NI-cRIO9022-019C2C95\\Mod6\\DO4"(w291) -> ()  [unwired: 1 in, 1 out]
                }
                frame "Flight Number" {
                  n233 = Variant To Data(error in=w300, type="", Variant=w298) -> (data=→"Flight Number":string, error out=w299:errorcluster)
                }
              }
            }
            frame True {
            }
          }
          n234 = node-c288() -> ()  [unwired: 1 in, 1 out]
        }
        n235 = node-c288(w249) -> ()  [unwired: 1 out]
        n236 = Destroy Stream Endpoint(8:w254, 11:w253) -> (0:→"error out":errorcluster)
        n237 = Wait (ms)(milliseconds to wait=u32 1000) -> ()  [unwired: 1 out]
      }
      n238 = while {
        tunnel: w44 -> [w67]
        tunnel: w45 -> [w66]
        stop <- w70 stop-if-true
        # "Must delay to avoid 100% CPU on cRIO"
        # "TCP Loop writing to SEPTIC Tank"
        n239 = TCP Open Connection(address="192.168.101.108", remote port or service name=u16 3502) -> (connection ID=w73:refnum<k5>, error out=w68:errorcluster)  [unwired: 3 in]
        n240 = case shown="No Error" w68 {
          selector: w68 -> [w78 w105]
          tunnel: w73 -> [w83 w106]
          tunnel: [w82 w106] -> w72
          tunnel: [w81 w105] -> w71
          tunnel: [w80 w104] -> w70
          tunnel: w66 -> [w77 _]
          tunnel: w67 -> [w76 _]
          frame No Error {
            n241 = node-c288() -> (w85:T1)  [unwired: 4 in]
            n242 = timed-loop {
              tunnel: w83 -> [w99]
              tunnel: w78 -> [w98]
              tunnel: [w97] -> w82
              tunnel: [w96] -> w81
              tunnel: [w86] -> w80
              shift-right: [w90] -> _
              shift-left: FALSE -> [w93]
              timing: w85 -> [_]
              timing-out: [_] -> w84
              tunnel: w77 -> [w89]
              tunnel: w76 -> [w88]
              stop <- w94 stop-if-true
              n243 = node-c288() -> ()  [unwired: 1 in, 1 out]
              n244 = Dequeue Element(queue=w89, error in (no error)=w88) -> (element=w87:string)  [unwired: 1 in, 3 out]
              n245 = Select(t=FALSE, s=w93, f=TRUE) -> (s? t:f=w90:bool)
              "TCP packet\nSend to SEPTIC" <- w90
              n246 = TCP Write(connection ID=w99, data in=w87, error in (no error)=w98) -> (connection ID out=w97:refnum<k5>, error out=w96:errorcluster)  [unwired: 1 in, 1 out]
              n247 = local read "stop"() -> (w86:bool)
              n248 = Unbundle(w96) -> ("status"=w95:bool)  [unwired: 2 out]
              n249 = node-c288() -> ()  [unwired: 1 in, 1 out]
              n250 = Compound Arithmetic op=OR(w95, w86) -> (w94:bool)
            }
            n251 = node-c288(w84) -> ()  [unwired: 1 out]
          }
          frame Error {
            n252 = local read "stop"() -> (w104:bool)
          }
        }
        n253 = TCP Close Connection(connection ID=w72, error in (no error)=w71) -> (error out=→"SEPTIC TCP Error Out":errorcluster)  [unwired: 1 in, 1 out]
        n254 = Wait (ms)(milliseconds to wait=u32 1000) -> ()  [unwired: 1 out]
      }
      n255 = while {
        tunnel: w53 -> [w109]
        tunnel: w52 -> [w108]
        stop <- w112 stop-if-true
        # "Must delay to avoid 100% CPU on cRIO"
        # "TCP Loop writing to FISH Tank"
        n256 = TCP Open Connection(address="192.168.101.110", remote port or service name=u16 3502) -> (connection ID=w115:refnum<k5>, error out=w110:errorcluster)  [unwired: 3 in]
        n257 = case shown="No Error" w110 {
          selector: w110 -> [w120 w147]
          tunnel: w115 -> [w125 w148]
          tunnel: [w124 w148] -> w114
          tunnel: [w123 w147] -> w113
          tunnel: [w122 w146] -> w112
          tunnel: w109 -> [w119 _]
          tunnel: w108 -> [w118 _]
          frame No Error {
            n258 = node-c288() -> (w127:T1)  [unwired: 4 in]
            n259 = timed-loop {
              tunnel: w125 -> [w141]
              tunnel: w120 -> [w140]
              tunnel: [w139] -> w124
              tunnel: [w138] -> w123
              tunnel: [w135] -> w122
              shift-right: [w131] -> _
              shift-left: FALSE -> [w134]
              timing: w127 -> [_]
              timing-out: [_] -> w126
              tunnel: w119 -> [w130]
              tunnel: w118 -> [w129]
              stop <- w136 stop-if-true
              n260 = node-c288() -> ()  [unwired: 1 in, 1 out]
              n261 = Dequeue Element(queue=w130, error in (no error)=w129) -> (element=w128:string)  [unwired: 1 in, 3 out]
              n262 = Select(t=FALSE, s=w134, f=TRUE) -> (s? t:f=w131:bool)
              "TCP packet\nSend to FISH" <- w131
              n263 = TCP Write(connection ID=w141, data in=w128, error in (no error)=w140) -> (connection ID out=w139:refnum<k5>, error out=w138:errorcluster)  [unwired: 1 in, 1 out]
              n264 = local read "stop"() -> (w135:bool)
              n265 = Unbundle(w138) -> ("status"=w137:bool)  [unwired: 2 out]
              n266 = node-c288() -> ()  [unwired: 1 in, 1 out]
              n267 = Compound Arithmetic op=OR(w137, w135) -> (w136:bool)
            }
            n268 = node-c288(w126) -> ()  [unwired: 1 out]
          }
          frame Error {
            n269 = local read "stop"() -> (w146:bool)
          }
        }
        n270 = TCP Close Connection(connection ID=w114, error in (no error)=w113) -> (error out=→"FISH TCP Error Out":errorcluster)  [unwired: 1 in, 1 out]
        n271 = Wait (ms)(milliseconds to wait=u32 1000) -> ()  [unwired: 1 out]
      }
      n272 = node-c288(w39) -> ()  [unwired: 1 out]
    }
    frame Error {
    }
  }
  n273 = VISA Close(VISA resource name=w22, error in (no error)=w21) -> (error out=→"Serial Visa Error":errorcluster)
